vi "KeyboardPress.vi"(8 "error in (no error)":errorcluster, 11 "View in":refnum<class "View.lvclass">) -> (0 "error out":errorcluster, 3 "View out":refnum<class "View.lvclass">)   [LabVIEW 2024, in "GUI.lvlib" / "View.lvclass"]
uses:
  View.lvclass
  View.lvclass/View.ctl
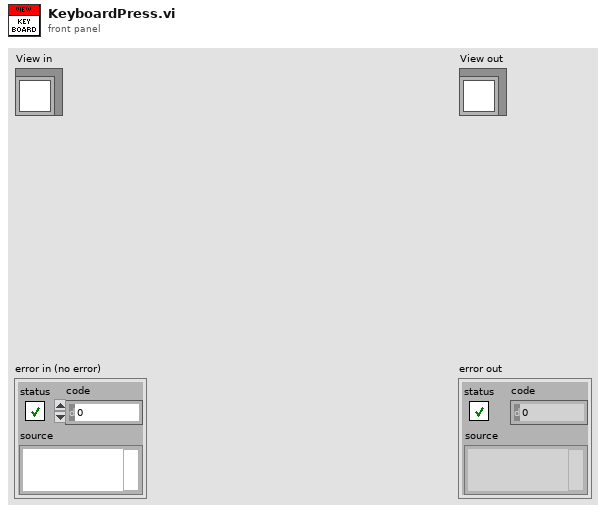
[diagram p1: front panel]
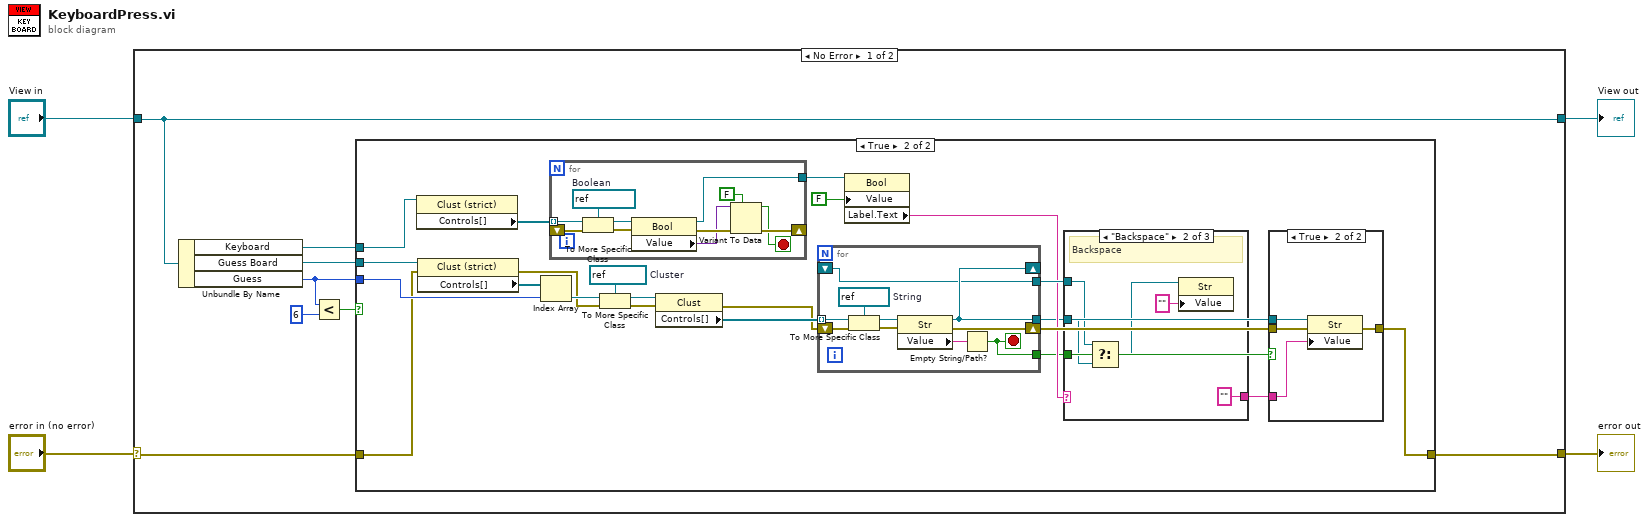
[diagram p0: block diagram]
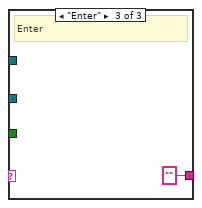
[diagram p5: hidden frame]
diagram:
  n1 = case shown="No Error" "error in (no error)" {
    selector: "error in (no error)" -> [w10 w71]
    tunnel: [w9 w71] -> w3
    tunnel: [w11 w70] -> w1
    tunnel: "View in" -> [w11 w70]
    frame No Error {
      n2 = Unbundle By Name(w11) -> ("Keyboard"=w8:refnum<vi>, "Guess Board"=w12:refnum<vi>, "Guess"=w6:i32)
      n3 = Less?(x=w6, y=6) -> (x < y?=w7:bool)
      n4 = case shown="True" w7 {
        tunnel: w12 -> [_ w35]
        tunnel: w6 -> [_ w33]
        tunnel: w10 -> [w13 w22]
        tunnel: [w13 w21] -> w9
        tunnel: w8 -> [_ w20]
        frame False {
        }
        frame True {
          w31 = refnum<vi> refnum  # Cluster
          n5 = property class="Clust (strict)"(reference=w20) -> ("Controls[]"=w19:refnum<vi>[])  [unwired: 1 in, 2 out]
          n6 = property class="Clust (strict)"(reference=w35, error in=w22) -> (error out=w27:errorcluster, "Controls[]"=w34:refnum<vi>[])  [unwired: 1 out]
          n7 = Index Array(array=w34, index=w33) -> (element=w32:refnum<vi>)
          n8 = for {
            tunnel: w19 -> [w45] mode=indexing
            shift-right: [w40] -> _
            shift-left: _ -> [w42]
            tunnel: [w36] -> w18
            stop <- w37 stop-if-true
            w46 = refnum<vi> refnum  # Boolean
            n9 = To More Specific Class(target class=w46, reference=w45, error in=w42) -> (specific class reference=w44:refnum<vi>, error out=w43:errorcluster)
            n10 = property class="Bool"(reference=w44, error in=w43) -> (reference out=w36:refnum<vi>, error out=w41:errorcluster, "Value"=w39:variant)
            n11 = Variant To Data(error in=w41, type=FALSE, Variant=w39) -> (data=w37:bool, error out=w40:errorcluster)
          }
          n12 = To More Specific Class(target class=w31, reference=w32, error in=w27) -> (specific class reference=w30:refnum<vi>, error out=w26:errorcluster)
          n13 = property class="Clust"(reference=w30, error in=w26) -> (error out=w25:errorcluster, "Controls[]"=w29:refnum<vi>[])  [unwired: 1 out]
          n14 = for {
            tunnel: w29 -> [w60] mode=indexing
            tunnel: [w54] -> w14
            shift-right: [w57] -> w24
            shift-left: w25 -> [w56]
            shift-right: [w54] -> _
            shift-left: _ -> [w53]
            tunnel: [w53] -> w23
            tunnel: [w52] -> w15
            stop <- w52 stop-if-true
            w61 = refnum<vi> refnum  # String
            n15 = To More Specific Class(target class=w61, reference=w60, error in=w56) -> (specific class reference=w59:refnum<vi>, error out=w55:errorcluster)
            n16 = property class="Str"(reference=w59, error in=w55) -> (reference out=w54:refnum<vi>, error out=w57:errorcluster, "Value"=w58:string)
            n17 = Empty String/Path?(string/path=w58) -> (empty?=w52:bool)
          }
          n18 = property class="Bool"(reference=w18, "Value"=FALSE) -> ("Label.Text"=w16:string)  [unwired: 1 in, 2 out]
          n19 = case shown="\"Backspace\"" w16 {
            selector: w16 -> [w62 _ _]
            tunnel: [w62 "" ""] -> w28
            tunnel: w23 -> [_ w65 _]
            tunnel: w15 -> [_ w66 _]
            tunnel: w14 -> [_ w64 _]
            frame Default {
            }
            frame "Backspace" {
              # "Backspace"
              n20 = Select(t=w65, s=w66, f=w64) -> (s? t:f=w63:refnum<vi>)
              n21 = property class="Str"(reference=w63, "Value"="") -> ()  [unwired: 1 in, 2 out]
            }
            frame "Enter" {
              # "Enter"
            }
          }
          n22 = case shown="True" w15 {
            tunnel: w14 -> [_ w51]
            tunnel: w28 -> [_ w50]
            tunnel: w24 -> [w47 w49]
            tunnel: [w47 w48] -> w21
            frame False {
            }
            frame True {
              n23 = property class="Str"(reference=w51, error in=w49, "Value"=w50) -> (error out=w48:errorcluster)  [unwired: 1 out]
            }
          }
        }
      }
    }
    frame Error {
    }
  }
  "error out" <- w3
  "View out" <- w1
